vi "final_control_mk6_022725.vi"() -> ()   [LabVIEW 2023]
doc: "Simplified example program for initializing the COM port, determining the data frame of up to 26 Alicats, acquiring the data of the same number of Alicats, displaying the data of the one with the selected unit ID, and writing a setpoint to the same selected unit ID.\n\nThis is a slightly more feature rich version of the Alicat Simplified Driver Example, and contains an example of a method for interfacing with up to 26 Alicats on a single COM port by means of for loops with shift registers to handle sequential commands to each included Alicat. This also contains a method to write a setpoint to the same selected unit.\n\nIf coding for multiple Alicats on a single COM port without the use of for loops with shift registers, ensure that each Alicat command is executed sequentially. Alicat's RS-232/485 does not work if multiple devices are responding simultaneously."
uses:
  <vilib>/Platform/TimedLoop/XDataNode/timing_clust.ctl
  <vilib>/Platform/TimedLoop/XDataNode/nitl_modes.ctl
  <vilib>/Platform/TimedLoop/XDataNode/wakeup.ctl
  <vilib>/DAQmx/write.llb/DAQmx Write (Analog 1D DBL NChan 1Samp).vi
  <extravilib>/ChannelInstances/Tag-bool/Read With Abort.vi
  <extravilib>/ChannelInstances/Tag-bool/Write With Abort.vi
  <vilib>/Utility/file.llb/Write Delimited Spreadsheet (string).vi
  <extravilib>/ChannelInstances/Tag-bool/Instantiate.vi
  <vilib>/Utility/file.llb/Read Delimited Spreadsheet (DBL).vi
  <extravilib>/ChannelInstances/Tag-bool/EndpointRead.vi
  <vilib>/DAQmx/miscellaneous.llb/DAQmx Fill In Error Info.vi
  <extravilib>/ChannelInstances/Tag-bool/Endpoint.vi
  <vilib>/platform/TimedLoop/XDataNode/XDataNode.xnode
  <vilib>/DAQmx/read.llb/DAQmx Read (Analog 1D DBL 1Chan NSamp).vi
  <vilib>/Platform/TimedLoop/XDataNode/XDNodeRunTimeDep.lvlib
  <extravilib>/ChannelInstances/Tag-bool.lvlib
panel:
  in  "Tab Control":enum32{"Page 1", "Page 2"}(tab)
  in  "COM Port Settings":T1={"Baud Rate"=enum."19200", "VISA Sesssion In"="MassFlowControllers"}
  out "Range Exceeded":bool
  out "Error Present":bool
  out "Error Text":string
  out "Elapsed Time [ms]\n(all units)":dbl caption="Elapsed Time (s)"
  in  "Minimum time between \nreadings [ms] (all units)":u32
  in  "Device ID's \nto Include:":T2={"A"=TRUE, "B"=TRUE, "C"=TRUE, "D"=TRUE, "E"=TRUE, "F"=TRUE, "G"=FALSE, "H"=FALSE, "I"=FALSE, "J"=FALSE, "K"=FALSE, "L"=FALSE, "M"=FALSE, "N"=FALSE, "O"=FALSE, "P"=FALSE, "Q"=FALSE, "R"=FALSE, "S"=FALSE, "T"=FALSE, "U"=FALSE, "V"=FALSE, "W"=FALSE, "X"=FALSE, "Y"=FALSE, "Z"=FALSE}
  out "Active Device":u16(ring) items=["A", "B", "C", "D", "E", "F"]
  out "Meas. Data (for active device)":T3
  in  "Write File":path
  in  "Hold Time [min]":dbl=17.0 min=17.0
  out "Global Start Time":i64
  out "N":i32
  out "Iteration Duration":i64
  in  "Read File":path
  in  "End Program":bool
  in  "Start From:":i32
  out "len_SP":i32
  out "Setpoints":dbl[][](array[numeric])=[[4.2, 3.3], [69.0, 4.2]]
  out "Z":dbl[](array[numeric])
  out "ASP":dbl
  out "BSP":dbl
  out "CSP":dbl
  out "DSP":dbl
  out "ESP":dbl
  out "FSP":dbl
  out "N_i_read":dbl
  out "N_read":i32
  out "read count":dbl=2.0
  out "T_SCh":string[](array[string])
  out "Iter_#":string
  out "V_D":string
  out "V_H":string
  out "Iter_Duration":string
  out "all rows":dbl[][](array[numeric])
  # "Totalizer Timer"
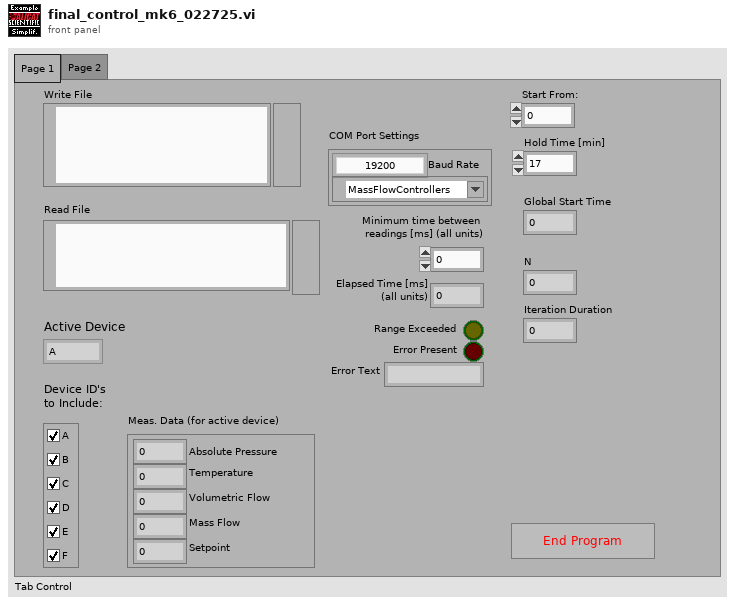
[diagram p1: front panel]
types:
  T1 = cluster{"Baud Rate":enum8{"2400", "9600", "19200", "38400", "57600", "115200", "Unknown"}, "VISA Sesssion In":refnum<visa-resource-name>}
  T2 = cluster{"A":bool, "B":bool, "C":bool, "D":bool, "E":bool, "F":bool, "G":bool, "H":bool, "I":bool, "J":bool, "K":bool, "L":bool, "M":bool, "N":bool, "O":bool, "P":bool, "Q":bool, "R":bool, "S":bool, "T":bool, "U":bool, "V":bool, "W":bool, "X":bool, "Y":bool, "Z":bool}
  T3 = cluster{"Absolute Pressure":dbl, "Gauge/Diff. Pressure":dbl, "Barometric Pressure":dbl, "Temperature":dbl, "Volumetric Flow":dbl, "Mass Flow":dbl, "Setpoint":dbl, "Valve Drive":dbl, "Totalizer":dbl, "[hr]":dbl, "[min]":dbl, "[sec]":dbl, "Totalizer Average Flow":dbl, "Totalizer Peak Flow":dbl, "Gas selected":string}
  T4 = cluster{"Unit ID":string, "Baud Rate":enum8{"2400", "9600", "19200", "38400", "57600", "115200", "Unknown"}, "VISA Sesssion In":refnum<visa-resource-name>}
  T5 = typedef "XDNodeRunTimeDep.lvlib/timing_clust.ctl" = cluster{"Expected End [f-1]":u64, "Actual End [f-1]":u64, "Finished Late? [f-1]":bool, "Expected End [i-1]":u64, "Actual End [i-1]":u64, "Finished Late? [i-1]":bool, "Expected Start [i]":u64, "Actual Start [i]":u64, "Expected Start [f]":u64, "Actual Start [f]":u64, "Source Name":string, "Structure Name":string, "Period":i64, "Deadline":i64, "Offset":i64, "Start":i64, "Priority":i32, "Timeout":i32, "Mode":T6, "Wakeup Reason":T7, "Error":errorcluster, "Source Type":string, "Secondary Source Type":string, "Global End Time":u64, "Global Start Time":u64, "Frame Duration":u64, "Iteration Duration":u64, "Assigned CPU":i32, "I/O Scan Engine Mode":u32}
  T6 = typedef "XDNodeRunTimeDep.lvlib/nitl_modes.ctl" = enum32{"No Change", "Process missed periods, maintain original phase", "Discard missed periods, maintain original phase", "Process missed periods, ignore original phase", "Discard missed periods, ignore original phase"}
  T7 = typedef "XDNodeRunTimeDep.lvlib/wakeup.ctl" = enum32{"Normal", "Aborted", "Asynchronous wakeup", "Timing source error", "Timed loop error", "Timeout"}
  T8 = typedef "Tag-bool.lvlib/))Channel.ctl" = refnum<queue>
  T9 = enum8{"2400", "9600", "19200", "38400", "57600", "115200", "Unknown"}
  T10 = cluster{"Absolute Pressure":bool, "Gauge/Diff. Pressure":bool, "Barometric Pressure":bool, "Temperature":bool, "Volumetric":bool, "Mass":bool, "Setpoint":bool, "Valve Drive":bool, "Totalizer":bool, "Totalizer Timer":bool, "Totalizer Average Flow":bool, "Totalizer Peak Flow":bool, "Gas Selected":bool, "Tot. Timer Format":u16}
  T11 = cluster{"Controller Full Scale":dbl, "Controller Select":u16, "Control Range":enum16{"Normal", "Inverted", "Bidirectional", "Unknown"}}
  T12 = cluster{"Controller Full Scale":dbl, "Controller Select":u16, "Control Range":enum16{"Normal", "Inverted", "Bidirectional", "Unknown"}}[]
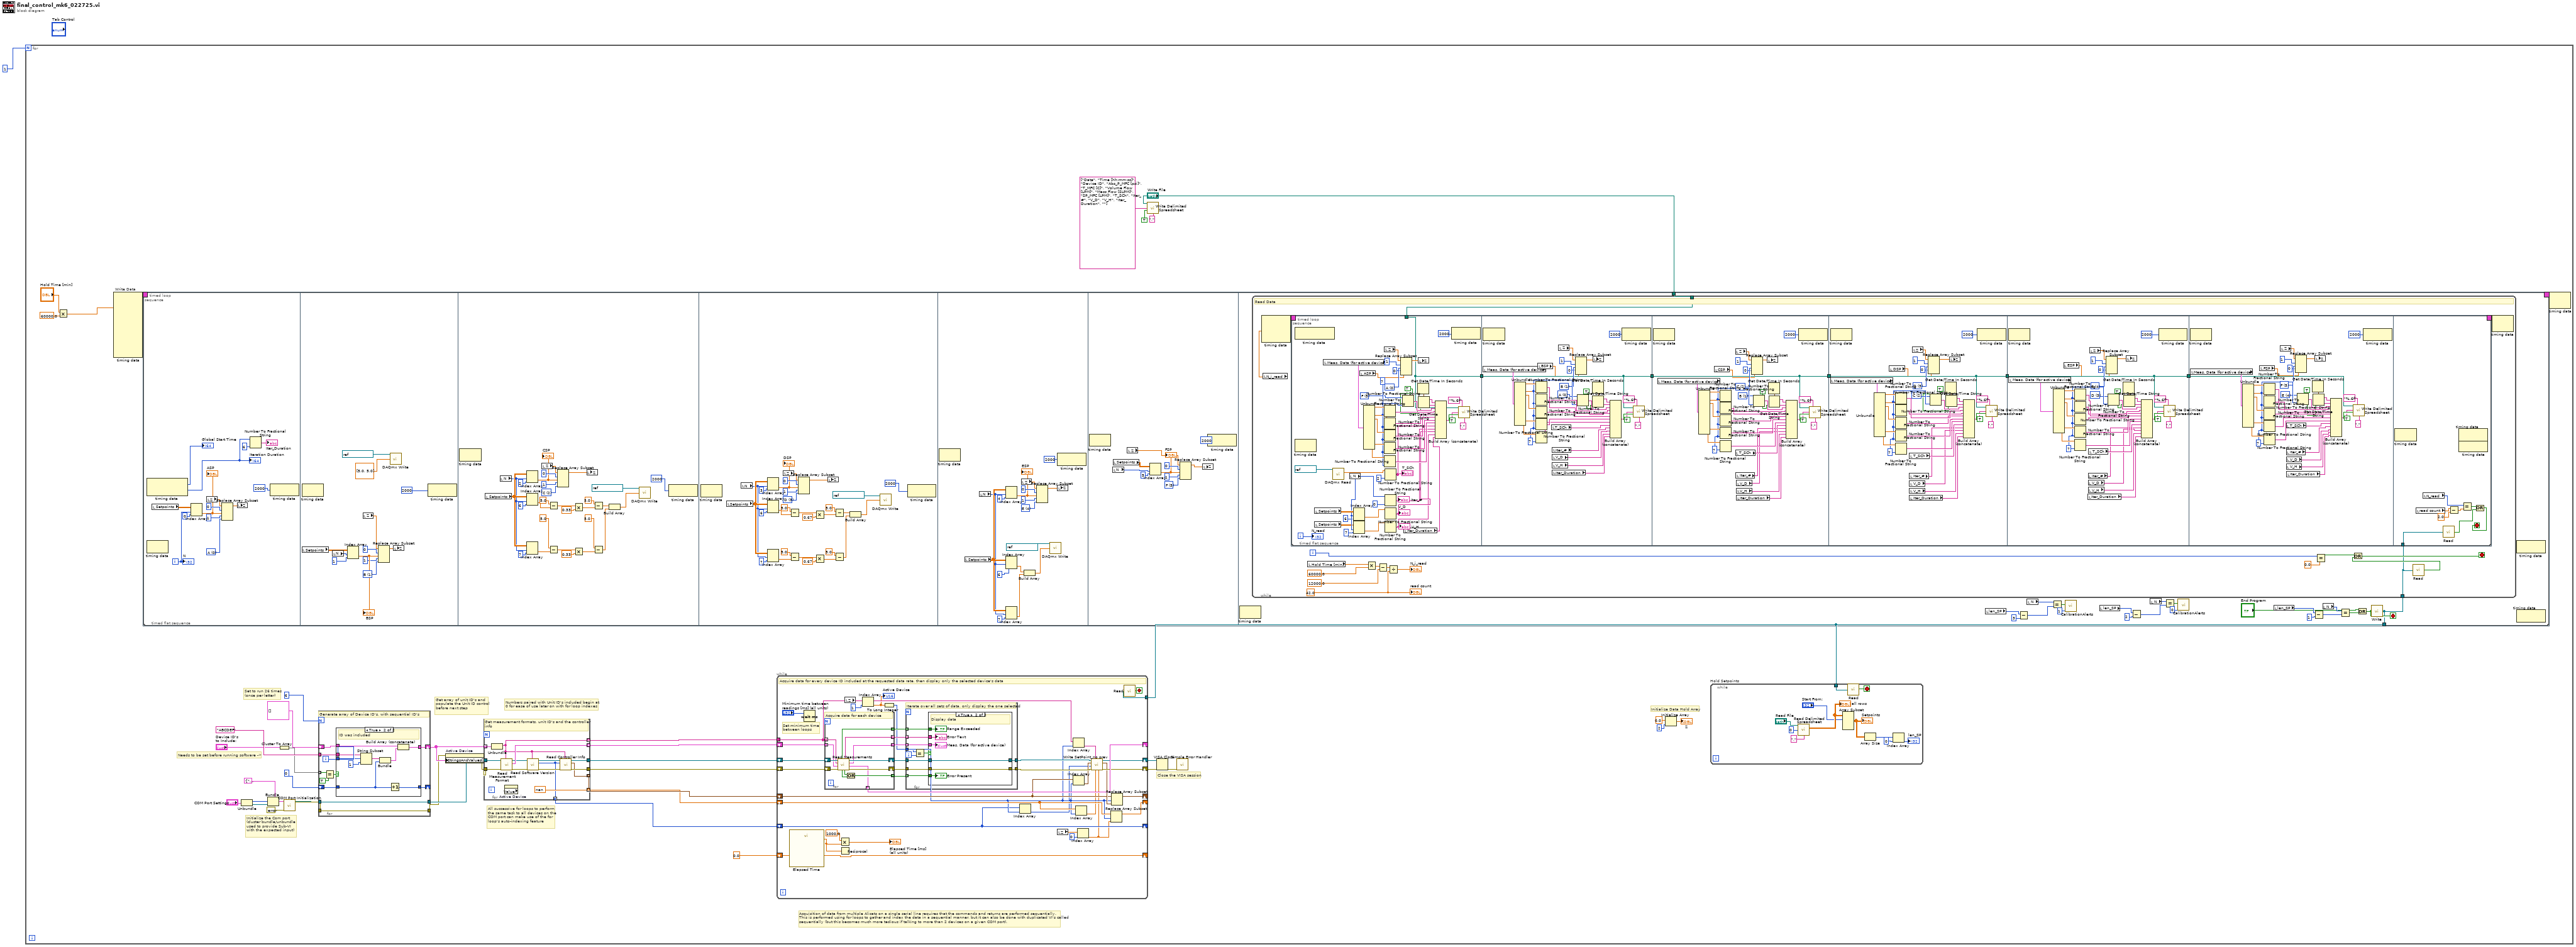
[diagram p0: block diagram]
diagram:
  n1 = for {
    N: 1 -> [_]
    # "Initialize Data Hold Array"
    # "All successive for loops to perform\nthe same task to all devices on the\nCOM port can make use of the for\nloop's auto-indexing feature"
    # "Set to run 26 times\n(once per letter)"
    # "Acquisition of data from multiple Alicats on a single serial line requires that the commands and returns are performed sequentially.\nThis is performed using for loops to gather and index the data in a sequential manner, but it can also be done with duplicated VI's called\nsequentially (but this becomes much more tedious if talking to more than 2 devices on a given COM port)."
    # "Numbers paired with Unit ID's included begin at\n0 for ease of use later on with for loop indexes"
    # "Get array of unit ID's and populate the Unit ID control before next step"
    # "Needs to be set before running software ->"
    # "Close the VISA session"
    # "Initialize the Com port\n(cluster bundle/unbundle\nused to provide Sub-VI \nwith the expected input)"
    n2 = Multiply(x="Hold Time [min]", y=60000.0) -> (x*y=w2:dbl)
    n3 = node-c288(w2) -> (w43:T5)  [unwired: 9 in]
    n4 = timed-loop "Write Data" {
      timing: w43 -> [_]
      timing-out: [_] -> w42
      tunnel: [w56] -> w9
      tunnel: "Write File" -> [w55]
      i -> [w70]
      stop <- w210 stop-if-true
      n5 = timed-sequence {
        timing: _ -> [_]
        timing-out: _ -> [_]
        tunnel: [w58] -> w56
        tunnel: w55 -> [w57]
        n6 = timed-flat-sequence {
          tunnel: [w205] -> w58
          tunnel: w57 -> [w206]
          frame #0 {
            w63 = u16 0 items=["A", "B", "C", "D", "E", "F"]
            n7 = node-c288() -> (→"Global Start Time":i64, w62:i64)  [unwired: 1 in]
            "Iteration Duration" <- w62
            n8 = local read "Setpoints"() -> (w72:dbl[][])
            n9 = Index Array(array=w72, index (row)=w70, index (col)=0 ("index (row)")) -> (element=w68:dbl)
            "ASP" <- w68
            n10 = local read "Z"() -> (w66:dbl[])
            n11 = Replace Array Subset(array=w66, new element #1=w68, index #1=0 ("index"), new element #2=w63, index #2=1 ("index")) -> (w67:dbl[])
            n12 = local write "Z"(w67) -> ()
            n13 = Number To Fractional String(number=w62, precision (6)=i16 6) -> (F-format string=→"Iter_Duration":string)  [unwired: 2 in]
            n14 = node-c288(i64 2000 ("Start")) -> ()  [unwired: 1 out]
            "N" <- w70
          }
          frame #1 {
            w81 = u16 1 items=["A", "B", "C", "D", "E", "F"]
            n15 = node-c288() -> ()  [unwired: 1 in, 1 out]
            n16 = local read "Setpoints"() -> (w89:dbl[][])
            n17 = local read "N"() -> (w82:i32)
            n18 = Index Array(array=w89, index (row)=w82, index (col)=1 ("index (row)")) -> (element=w86:dbl)
            "BSP" <- w86
            n19 = local read "Z"() -> (w84:dbl[])
            n20 = Replace Array Subset(array=w84, new element #1=w86, index #1=0 ("index"), new element #2=w81, index #2=1 ("index")) -> (w85:dbl[])
            n21 = call-poly <vilib>:"DAQmx Write.vi"("task/channels in"=refnum<k21> "Valve_cont", "data"=dbl[] [5.0, 5.0]) -> ()  [unwired: 11 in, 3 out]
            n22 = local write "Z"(w85) -> ()
            n23 = node-c288(i64 2000 ("Start")) -> ()  [unwired: 1 out]
          }
          frame #2 {
            w115 = u16 2 items=["A", "B", "C", "D", "E", "F"]
            n24 = node-c288() -> ()  [unwired: 1 in, 1 out]
            n25 = local read "Setpoints"() -> (w98:dbl[][])
            n26 = local read "N"() -> (w97:i32)
            n27 = Index Array(array=w98, index (row)=w97, index (col)=2 ("index (row)")) -> (element=w119:dbl)
            "CSP" <- w119
            n28 = Index Array(array=w98, index (row)=w97, index (col)=6 ("disabled index (col)")) -> (element=w96:dbl)
            n29 = Index Array(array=w98, index (row)=w97, index (col)=7 ("disabled index (col)")) -> (element=w95:dbl)
            n30 = local read "Z"() -> (w117:dbl[])
            n31 = Subtract(x=5.0, y=w96) -> (x-y=w112:dbl)
            n32 = Subtract(x=5.0, y=w95) -> (x-y=w107:dbl)
            n33 = Replace Array Subset(array=w117, new element #1=w119, index #1=0 ("index"), new element #2=w115, index #2=1 ("index")) -> (w118:dbl[])
            n34 = Multiply(x=w112, y=0.33) -> (x*y=w110:dbl)
            n35 = Multiply(x=w107, y=0.33) -> (x*y=w105:dbl)
            n36 = local write "Z"(w118) -> ()
            n37 = Subtract(x=5.0, y=w110) -> (x-y=w100:dbl)
            n38 = Subtract(x=5.0, y=w105) -> (x-y=w101:dbl)
            n39 = Build Array(w100, w101) -> (w99:dbl[])
            n40 = call-poly <vilib>:"DAQmx Write.vi"("task/channels in"=refnum<k21> "Valve_cont", "data"=w99) -> ()  [unwired: 11 in, 3 out]
            n41 = node-c288(i64 2000 ("Start")) -> ()  [unwired: 1 out]
          }
          frame #3 {
            w147 = u16 3 items=["A", "B", "C", "D", "E", "F"]
            n42 = node-c288() -> ()  [unwired: 1 in, 1 out]
            n43 = local read "Setpoints"() -> (w130:dbl[][])
            n44 = local read "N"() -> (w129:i32)
            n45 = Index Array(array=w130, index (row)=w129, index (col)=3 ("index (row)")) -> (element=w151:dbl)
            "DSP" <- w151
            n46 = Index Array(array=w130, index (row)=w129, index (col)=6 ("disabled index (col)")) -> (element=w128:dbl)
            n47 = Index Array(array=w130, index (row)=w129, index (col)=7 ("disabled index (col)")) -> (element=w127:dbl)
            n48 = local read "Z"() -> (w149:dbl[])
            n49 = Subtract(x=5.0, y=w128) -> (x-y=w144:dbl)
            n50 = Subtract(x=5.0, y=w127) -> (x-y=w139:dbl)
            n51 = Replace Array Subset(array=w149, new element #1=w151, index #1=0 ("index"), new element #2=w147, index #2=1 ("index")) -> (w150:dbl[])
            n52 = Multiply(x=w144, y=0.67) -> (x*y=w142:dbl)
            n53 = Multiply(x=w139, y=0.67) -> (x*y=w137:dbl)
            n54 = local write "Z"(w150) -> ()
            n55 = Subtract(x=5.0, y=w142) -> (x-y=w132:dbl)
            n56 = Subtract(x=5.0, y=w137) -> (x-y=w133:dbl)
            n57 = Build Array(w132, w133) -> (w131:dbl[])
            n58 = call-poly <vilib>:"DAQmx Write.vi"("task/channels in"=refnum<k21> "Valve_cont", "data"=w131) -> ()  [unwired: 11 in, 3 out]
            n59 = node-c288(i64 2000 ("Start")) -> ()  [unwired: 1 out]
          }
          frame #4 {
            w168 = u16 4 items=["A", "B", "C", "D", "E", "F"]
            n60 = node-c288() -> ()  [unwired: 1 in, 1 out]
            n61 = local read "Setpoints"() -> (w162:dbl[][])
            n62 = local read "N"() -> (w161:i32)
            n63 = Index Array(array=w162, index (row)=w161, index (col)=4 ("index (row)")) -> (element=w172:dbl)
            "ESP" <- w172
            n64 = Index Array(array=w162, index (row)=w161, index (col)=6 ("disabled index (col)")) -> (element=w164:dbl)
            n65 = Index Array(array=w162, index (row)=w161, index (col)=7 ("disabled index (col)")) -> (element=w163:dbl)
            n66 = local read "Z"() -> (w170:dbl[])
            n67 = Build Array(w164, w163) -> (w160:dbl[])
            n68 = Replace Array Subset(array=w170, new element #1=w172, index #1=0 ("index"), new element #2=w168, index #2=1 ("index")) -> (w171:dbl[])
            n69 = call-poly <vilib>:"DAQmx Write.vi"("task/channels in"=refnum<k21> "Valve_cont", "data"=w160) -> ()  [unwired: 11 in, 3 out]
            n70 = local write "Z"(w171) -> ()
            n71 = node-c288(i64 2000 ("Start")) -> ()  [unwired: 1 out]
          }
          frame #5 {
            w182 = u16 5 items=["A", "B", "C", "D", "E", "F"]
            n72 = node-c288() -> ()  [unwired: 1 in, 1 out]
            n73 = local read "N"() -> (w180:i32)
            n74 = local read "Setpoints"() -> (w185:dbl[][])
            n75 = local read "Z"() -> (w184:dbl[])
            n76 = Index Array(array=w185, index (row)=w180, index (col)=5 ("index (row)")) -> (element=w181:dbl)
            "FSP" <- w181
            n77 = Replace Array Subset(array=w184, new element #1=w181, index #1=0 ("index"), new element #2=w182, index #2=1 ("index")) -> (w183:dbl[])
            n78 = local write "Z"(w183) -> ()
            n79 = node-c288(i64 2000 ("Start")) -> ()  [unwired: 1 out]
          }
          frame #6 {
            n80 = node-c288() -> ()  [unwired: 1 in, 1 out]
            n81 = local read "len_SP"() -> (w194:i32)
            n82 = Subtract(x=w194, y=3) -> (x-y=w196:i32)
            n83 = local read "N"() -> (w195:i32)
            n84 = Equal?(x=w195, y=w196) -> (x = y?=w197:bool)
            n85 = call "CalibrationAlerts.vi"("Alert Type (0)"=1, "Trigger"=w197) -> ()  [unwired: 10 in]
            n86 = local read "len_SP"() -> (w200:i32)
            n87 = Subtract(x=w200, y=2) -> (x-y=w199:i32)
            n88 = local read "N"() -> (w204:i32)
            n89 = Equal?(x=w204, y=w199) -> (x = y?=w202:bool)
            n90 = call "CalibrationAlerts.vi"("Alert Type (0)"=0, "Trigger"=w202) -> ()  [unwired: 10 in]
            n91 = local read "len_SP"() -> (w209:i32)
            n92 = Subtract(x=w209, y=1) -> (x-y=w212:i32)
            n93 = local read "N"() -> (w208:i32)
            n94 = Equal?(x=w208, y=w212) -> (x = y?=w211:bool)
            n95 = Or(x="End Program", y=w211) -> (x .or. y?=w210:bool)
            n96 = call <extravilib>:"Write.vi"("element"=w210) -> ("channel"=w205:T8)  [unwired: 1 out]
            n97 = while {
              tunnel: w206 -> [w228]
              tunnel: w205 -> [w214]
              i -> [w224]
              stop <- w223 stop-if-true
              w217 = 42.0 ("y")
              # "Read Data"
              n98 = local read "N_i_read"() -> (w222:dbl)
              n99 = node-c288(w222) -> (w230:T5)  [unwired: 2 in]
              n100 = timed-loop {
                timing: w230 -> [_]
                timing-out: [_] -> w229
                tunnel: w228 -> [w232]
                tunnel: w214 -> [w231]
                i -> [w258]
                stop <- w487 stop-if-true
                n101 = timed-sequence {
                  timing: _ -> [_]
                  timing-out: _ -> [_]
                  tunnel: w232 -> [w239]
                  tunnel: w231 -> [w233]
                  n102 = timed-flat-sequence {
                    tunnel: w239 -> [w261]
                    tunnel: [w261] -> w238
                    tunnel: w238 -> [w300]
                    tunnel: [w300] -> w237
                    tunnel: w237 -> [w339]
                    tunnel: [w339] -> w236
                    tunnel: w236 -> [w378]
                    tunnel: [w378] -> w235
                    tunnel: w235 -> [w417]
                    tunnel: [w417] -> w234
                    tunnel: w234 -> [w457]
                    tunnel: w233 -> [w489]
                    frame #0 {
                      w257 = u16 5 items=["A", "B", "C", "D", "E", "F"]
                      w264 = u16 0 items=["A", "B", "C", "D", "E", "F"]
                      w265 = i16 7 ("precision (6)")
                      n103 = node-c288() -> ()  [unwired: 1 in, 1 out]
                      n104 = local read "Setpoints"() -> (w251:dbl[][])
                      n105 = local read "Setpoints"() -> (w247:dbl[][])
                      n106 = local read "Meas. Data (for active device)"() -> (w272:T3)
                      n107 = call-poly <vilib>:"DAQmx Read.vi"("task/channels in"=refnum<k21> "T_SCh") -> ("data"=w255:dbl[])  [unwired: 12 in, 2 out]
                      n108 = local read "N"() -> (w248:i32)
                      n109 = Index Array(array=w251, index (row)=w248, index (col)=6 ("disabled index (col)")) -> (element=w250:dbl)
                      n110 = Index Array(array=w247, index (row)=w248, index (col)=7 ("disabled index (col)")) -> (element=w249:dbl)
                      n111 = local read "ASP"() -> (w259:dbl)
                      n112 = Unbundle(w272) -> ("Absolute Pressure"=w285:dbl, "Temperature"=w281:dbl, "Volumetric Flow"=w271:dbl, "Mass Flow"=w282:dbl, "Setpoint"=w283:dbl)  [unwired: 10 out]
                      n113 = local read "Z"() -> (w268:dbl[])
                      n114 = Number To Fractional String(number=w285, precision (6)=w265) -> (F-format string=w280:string)  [unwired: 2 in]
                      n115 = Number To Fractional String(number=w281, precision (6)=w265) -> (F-format string=w279:string)  [unwired: 2 in]
                      n116 = Number To Fractional String(number=w271, precision (6)=w265) -> (F-format string=w278:string)  [unwired: 2 in]
                      n117 = Number To Fractional String(number=w282, precision (6)=w265) -> (F-format string=w277:string)  [unwired: 2 in]
                      n118 = Number To Fractional String(number=w283, precision (6)=w265) -> (F-format string=w276:string)  [unwired: 2 in]
                      n119 = Number To Fractional String(number=w255, precision (6)=i16 2) -> (F-format string=w254:string[])  [unwired: 2 in]
                      "T_SCh" <- w254
                      n120 = Number To Fractional String(number=w248, precision (6)=i16 0) -> (F-format string=w243:string)  [unwired: 2 in]
                      "Iter_#" <- w243
                      n121 = Number To Fractional String(number=w250) -> (F-format string=w242:string)  [unwired: 3 in]
                      "V_D" <- w242
                      n122 = Number To Fractional String(number=w249) -> (F-format string=w241:string)  [unwired: 3 in]
                      "V_H" <- w241
                      n123 = Replace Array Subset(array=w268, new element #1=w264, index #1=1 ("index"), new element #2=w259, index #2=0 ("index")) -> (w266:dbl[])
                      n124 = Number To Fractional String(number=w257, precision (6)=w265) -> (F-format string=w284:string)  [unwired: 2 in]
                      n125 = local read "Iter_Duration"() -> (w240:string)
                      n126 = Get Date/Time In Seconds() -> (seconds since 1Jan1904=w270:timestamp)
                      n127 = Get Date/Time String(seconds (now)=w270, want seconds? (F)=TRUE) -> (date string=w269:string, time string=w286:string)  [unwired: 1 in]
                      n128 = local write "Z"(w266) -> ()
                      n129 = Build Array (concatenate)(w269, w286, w284, w280, w279, w278, w277, w276, w254, w243, w242, w241, w240) -> (w273:string[])
                      n130 = node-c288(i64 2000 ("Start")) -> ()  [unwired: 1 out]
                      n131 = call-poly <vilib>:"Write Delimited Spreadsheet.vi"("file path (dialog if empty)"=w261, "format (%s)"="%.6f" ("format (%.3f)"), "1D data"=w273, "append to file? (new file:F)"=TRUE, "delimiter (\\t)"="," ("delimiter (\\t)")) -> ()  [unwired: 9 in, 2 out]
                      "N_read" <- w258
                    }
                    frame #1 {
                      w297 = u16 0 items=["A", "B", "C", "D", "E", "F"]
                      w306 = u16 1 items=["A", "B", "C", "D", "E", "F"]
                      w307 = i16 7 ("precision (6)")
                      n132 = node-c288() -> ()  [unwired: 1 in, 1 out]
                      n133 = local read "Meas. Data (for active device)"() -> (w304:T3)
                      n134 = Unbundle(w304) -> ("Absolute Pressure"=w324:dbl, "Temperature"=w320:dbl, "Volumetric Flow"=w311:dbl, "Mass Flow"=w321:dbl, "Setpoint"=w322:dbl)  [unwired: 10 out]
                      n135 = Number To Fractional String(number=w324, precision (6)=w307) -> (F-format string=w319:string)  [unwired: 2 in]
                      n136 = Number To Fractional String(number=w320, precision (6)=w307) -> (F-format string=w318:string)  [unwired: 2 in]
                      n137 = Number To Fractional String(number=w311, precision (6)=w307) -> (F-format string=w317:string)  [unwired: 2 in]
                      n138 = Number To Fractional String(number=w321, precision (6)=w307) -> (F-format string=w316:string)  [unwired: 2 in]
                      n139 = Number To Fractional String(number=w322, precision (6)=w307) -> (F-format string=w315:string)  [unwired: 2 in]
                      n140 = local read "BSP"() -> (w298:dbl)
                      n141 = local read "T_SCh"() -> (w296:string[])
                      n142 = local read "Iter_#"() -> (w294:string)
                      n143 = local read "V_D"() -> (w293:string)
                      n144 = local read "V_H"() -> (w292:string)
                      n145 = local read "Iter_Duration"() -> (w291:string)
                      n146 = local read "Z"() -> (w303:dbl[])
                      n147 = Replace Array Subset(array=w303, new element #1=w306, index #1=1 ("index"), new element #2=w298, index #2=0 ("index")) -> (w302:dbl[])
                      n148 = Number To Fractional String(number=w297, precision (6)=w307) -> (F-format string=w323:string)  [unwired: 2 in]
                      n149 = Get Date/Time In Seconds() -> (seconds since 1Jan1904=w310:timestamp)
                      n150 = Get Date/Time String(seconds (now)=w310, want seconds? (F)=TRUE) -> (date string=w309:string, time string=w325:string)  [unwired: 1 in]
                      n151 = local write "Z"(w302) -> ()
                      n152 = Build Array (concatenate)(w309, w325, w323, w319, w318, w317, w316, w315, w296, w294, w293, w292, w291) -> (w312:string[])
                      n153 = node-c288(i64 2000 ("Start")) -> ()  [unwired: 1 out]
                      n154 = call-poly <vilib>:"Write Delimited Spreadsheet.vi"("file path (dialog if empty)"=w300, "format (%s)"="%.6f" ("format (%.3f)"), "1D data"=w312, "append to file? (new file:F)"=TRUE, "delimiter (\\t)"="," ("delimiter (\\t)")) -> ()  [unwired: 9 in, 2 out]
                    }
                    frame #2 {
                      w336 = u16 1 items=["A", "B", "C", "D", "E", "F"]
                      w345 = u16 2 items=["A", "B", "C", "D", "E", "F"]
                      w346 = i16 7 ("precision (6)")
                      n155 = node-c288() -> ()  [unwired: 1 in, 1 out]
                      n156 = local read "Meas. Data (for active device)"() -> (w341:T3)
                      n157 = Unbundle(w341) -> ("Absolute Pressure"=w363:dbl, "Temperature"=w359:dbl, "Volumetric Flow"=w350:dbl, "Mass Flow"=w360:dbl, "Setpoint"=w361:dbl)  [unwired: 10 out]
                      n158 = local read "CSP"() -> (w337:dbl)
                      n159 = Number To Fractional String(number=w363, precision (6)=w346) -> (F-format string=w358:string)  [unwired: 2 in]
                      n160 = Number To Fractional String(number=w359, precision (6)=w346) -> (F-format string=w357:string)  [unwired: 2 in]
                      n161 = Number To Fractional String(number=w350, precision (6)=w346) -> (F-format string=w356:string)  [unwired: 2 in]
                      n162 = Number To Fractional String(number=w360, precision (6)=w346) -> (F-format string=w355:string)  [unwired: 2 in]
                      n163 = Number To Fractional String(number=w361, precision (6)=w346) -> (F-format string=w354:string)  [unwired: 2 in]
                      n164 = local read "Z"() -> (w343:dbl[])
                      n165 = local read "T_SCh"() -> (w335:string[])
                      n166 = local read "Iter_#"() -> (w333:string)
                      n167 = local read "V_D"() -> (w332:string)
                      n168 = local read "V_H"() -> (w331:string)
                      n169 = local read "Iter_Duration"() -> (w330:string)
                      n170 = Replace Array Subset(array=w343, new element #1=w345, index #1=1 ("index"), new element #2=w337, index #2=0 ("index")) -> (w342:dbl[])
                      n171 = Number To Fractional String(number=w336, precision (6)=w346) -> (F-format string=w362:string)  [unwired: 2 in]
                      n172 = local write "Z"(w342) -> ()
                      n173 = Get Date/Time In Seconds() -> (seconds since 1Jan1904=w349:timestamp)
                      n174 = Get Date/Time String(seconds (now)=w349, want seconds? (F)=TRUE) -> (date string=w348:string, time string=w364:string)  [unwired: 1 in]
                      n175 = Build Array (concatenate)(w348, w364, w362, w358, w357, w356, w355, w354, w335, w333, w332, w331, w330) -> (w351:string[])
                      n176 = node-c288(i64 2000 ("Start")) -> ()  [unwired: 1 out]
                      n177 = call-poly <vilib>:"Write Delimited Spreadsheet.vi"("file path (dialog if empty)"=w339, "format (%s)"="%.6f" ("format (%.3f)"), "1D data"=w351, "append to file? (new file:F)"=TRUE, "delimiter (\\t)"="," ("delimiter (\\t)")) -> ()  [unwired: 9 in, 2 out]
                    }
                    frame #3 {
                      w375 = u16 2 items=["A", "B", "C", "D", "E", "F"]
                      w384 = u16 3 items=["A", "B", "C", "D", "E", "F"]
                      w385 = i16 7 ("precision (6)")
                      n178 = node-c288() -> ()  [unwired: 1 in, 1 out]
                      n179 = local read "Meas. Data (for active device)"() -> (w382:T3)
                      n180 = Unbundle(w382) -> ("Absolute Pressure"=w402:dbl, "Temperature"=w398:dbl, "Volumetric Flow"=w389:dbl, "Mass Flow"=w399:dbl, "Setpoint"=w400:dbl)  [unwired: 10 out]
                      n181 = local read "DSP"() -> (w376:dbl)
                      n182 = Number To Fractional String(number=w402, precision (6)=w385) -> (F-format string=w397:string)  [unwired: 2 in]
                      n183 = Number To Fractional String(number=w398, precision (6)=w385) -> (F-format string=w396:string)  [unwired: 2 in]
                      n184 = Number To Fractional String(number=w389, precision (6)=w385) -> (F-format string=w395:string)  [unwired: 2 in]
                      n185 = Number To Fractional String(number=w399, precision (6)=w385) -> (F-format string=w394:string)  [unwired: 2 in]
                      n186 = Number To Fractional String(number=w400, precision (6)=w385) -> (F-format string=w393:string)  [unwired: 2 in]
                      n187 = local read "T_SCh"() -> (w374:string[])
                      n188 = local read "Iter_#"() -> (w372:string)
                      n189 = local read "V_D"() -> (w371:string)
                      n190 = local read "V_H"() -> (w370:string)
                      n191 = local read "Iter_Duration"() -> (w369:string)
                      n192 = local read "Z"() -> (w381:dbl[])
                      n193 = Replace Array Subset(array=w381, new element #1=w384, index #1=1 ("index"), new element #2=w376, index #2=0 ("index")) -> (w380:dbl[])
                      n194 = Number To Fractional String(number=w375, precision (6)=w385) -> (F-format string=w401:string)  [unwired: 2 in]
                      n195 = Get Date/Time In Seconds() -> (seconds since 1Jan1904=w388:timestamp)
                      n196 = Get Date/Time String(seconds (now)=w388, want seconds? (F)=TRUE) -> (date string=w387:string, time string=w403:string)  [unwired: 1 in]
                      n197 = local write "Z"(w380) -> ()
                      n198 = Build Array (concatenate)(w387, w403, w401, w397, w396, w395, w394, w393, w374, w372, w371, w370, w369) -> (w390:string[])
                      n199 = node-c288(i64 2000 ("Start")) -> ()  [unwired: 1 out]
                      n200 = call-poly <vilib>:"Write Delimited Spreadsheet.vi"("file path (dialog if empty)"=w378, "format (%s)"="%.6f" ("format (%.3f)"), "1D data"=w390, "append to file? (new file:F)"=TRUE, "delimiter (\\t)"="," ("delimiter (\\t)")) -> ()  [unwired: 9 in, 2 out]
                    }
                    frame #4 {
                      w414 = u16 3 items=["A", "B", "C", "D", "E", "F"]
                      w423 = u16 4 items=["A", "B", "C", "D", "E", "F"]
                      w424 = i16 7 ("precision (6)")
                      n201 = node-c288() -> ()  [unwired: 1 in, 1 out]
                      n202 = local read "Meas. Data (for active device)"() -> (w421:T3)
                      n203 = Unbundle(w421) -> ("Absolute Pressure"=w441:dbl, "Temperature"=w437:dbl, "Volumetric Flow"=w428:dbl, "Mass Flow"=w438:dbl, "Setpoint"=w439:dbl)  [unwired: 10 out]
                      n204 = local read "ESP"() -> (w415:dbl)
                      n205 = Number To Fractional String(number=w441, precision (6)=w424) -> (F-format string=w436:string)  [unwired: 2 in]
                      n206 = Number To Fractional String(number=w437, precision (6)=w424) -> (F-format string=w435:string)  [unwired: 2 in]
                      n207 = Number To Fractional String(number=w428, precision (6)=w424) -> (F-format string=w434:string)  [unwired: 2 in]
                      n208 = Number To Fractional String(number=w438, precision (6)=w424) -> (F-format string=w433:string)  [unwired: 2 in]
                      n209 = Number To Fractional String(number=w439, precision (6)=w424) -> (F-format string=w432:string)  [unwired: 2 in]
                      n210 = local read "Iter_Duration"() -> (w408:string)
                      n211 = local read "Iter_#"() -> (w411:string)
                      n212 = local read "V_D"() -> (w410:string)
                      n213 = local read "V_H"() -> (w409:string)
                      n214 = local read "T_SCh"() -> (w413:string[])
                      n215 = local read "Z"() -> (w420:dbl[])
                      n216 = Replace Array Subset(array=w420, new element #1=w423, index #1=1 ("index"), new element #2=w415, index #2=0 ("index")) -> (w419:dbl[])
                      n217 = Number To Fractional String(number=w414, precision (6)=w424) -> (F-format string=w440:string)  [unwired: 2 in]
                      n218 = Get Date/Time In Seconds() -> (seconds since 1Jan1904=w427:timestamp)
                      n219 = Get Date/Time String(seconds (now)=w427, want seconds? (F)=TRUE) -> (date string=w426:string, time string=w442:string)  [unwired: 1 in]
                      n220 = local write "Z"(w419) -> ()
                      n221 = Build Array (concatenate)(w426, w442, w440, w436, w435, w434, w433, w432, w413, w411, w410, w409, w408) -> (w429:string[])
                      n222 = node-c288(i64 2000 ("Start")) -> ()  [unwired: 1 out]
                      n223 = call-poly <vilib>:"Write Delimited Spreadsheet.vi"("file path (dialog if empty)"=w417, "format (%s)"="%.6f" ("format (%.3f)"), "1D data"=w429, "append to file? (new file:F)"=TRUE, "delimiter (\\t)"="," ("delimiter (\\t)")) -> ()  [unwired: 9 in, 2 out]
                    }
                    frame #5 {
                      w454 = u16 4 items=["A", "B", "C", "D", "E", "F"]
                      w462 = u16 5 items=["A", "B", "C", "D", "E", "F"]
                      w463 = i16 7 ("precision (6)")
                      n224 = node-c288() -> ()  [unwired: 1 in, 1 out]
                      n225 = local read "Meas. Data (for active device)"() -> (w460:T3)
                      n226 = Unbundle(w460) -> ("Absolute Pressure"=w480:dbl, "Temperature"=w476:dbl, "Volumetric Flow"=w467:dbl, "Mass Flow"=w477:dbl, "Setpoint"=w478:dbl)  [unwired: 10 out]
                      n227 = local read "FSP"() -> (w455:dbl)
                      n228 = Number To Fractional String(number=w480, precision (6)=w463) -> (F-format string=w475:string)  [unwired: 2 in]
                      n229 = Number To Fractional String(number=w476, precision (6)=w463) -> (F-format string=w474:string)  [unwired: 2 in]
                      n230 = Number To Fractional String(number=w467, precision (6)=w463) -> (F-format string=w473:string)  [unwired: 2 in]
                      n231 = Number To Fractional String(number=w477, precision (6)=w463) -> (F-format string=w472:string)  [unwired: 2 in]
                      n232 = Number To Fractional String(number=w478, precision (6)=w463) -> (F-format string=w471:string)  [unwired: 2 in]
                      n233 = local read "Z"() -> (w459:dbl[])
                      n234 = local read "T_SCh"() -> (w453:string[])
                      n235 = local read "Iter_#"() -> (w451:string)
                      n236 = local read "V_D"() -> (w450:string)
                      n237 = local read "V_H"() -> (w449:string)
                      n238 = local read "Iter_Duration"() -> (w448:string)
                      n239 = Replace Array Subset(array=w459, new element #1=w462, index #1=1 ("index"), new element #2=w455, index #2=0 ("index")) -> (w458:dbl[])
                      n240 = Number To Fractional String(number=w454, precision (6)=w463) -> (F-format string=w479:string)  [unwired: 2 in]
                      n241 = Get Date/Time In Seconds() -> (seconds since 1Jan1904=w466:timestamp)
                      n242 = Get Date/Time String(seconds (now)=w466, want seconds? (F)=TRUE) -> (date string=w465:string, time string=w481:string)  [unwired: 1 in]
                      n243 = local write "Z"(w458) -> ()
                      n244 = Build Array (concatenate)(w465, w481, w479, w475, w474, w473, w472, w471, w453, w451, w450, w449, w448) -> (w468:string[])
                      n245 = call-poly <vilib>:"Write Delimited Spreadsheet.vi"("file path (dialog if empty)"=w457, "format (%s)"="%.6f" ("format (%.3f)"), "1D data"=w468, "append to file? (new file:F)"=TRUE, "delimiter (\\t)"="," ("delimiter (\\t)")) -> ()  [unwired: 9 in, 2 out]
                      n246 = node-c288(i64 2000 ("Start")) -> ()  [unwired: 1 out]
                    }
                    frame #6 {
                      n247 = node-c288() -> ()  [unwired: 1 in, 1 out]
                      n248 = local read "read count"() -> (w493:dbl)
                      n249 = local read "N_read"() -> (w491:i32)
                      n250 = call <extravilib>:"Read.vi"("channel"=w489) -> ("element"=w488:bool)  [unwired: 1 in, 1 out]
                      n251 = Subtract(x=w493, y=2.0) -> (x-y=w492:dbl)
                      n252 = node-c288() -> ()  [unwired: 1 in, 1 out]
                      n253 = Equal?(x=w491, y=w492) -> (x = y?=w490:bool)
                      n254 = Or(x=w490, y=w488) -> (x .or. y?=w487:bool)
                    }
                  }
                }
                n255 = node-c288() -> ()  [unwired: 1 in, 1 out]
                n256 = node-c288() -> ()  [unwired: 1 in, 1 out]
              }
              n257 = local read "Hold Time [min]"() -> (w220:dbl)
              n258 = Multiply(x=w220, y=60000.0) -> (x*y=w219:dbl)
              n259 = Subtract(x=w219, y=12000.0) -> (x-y=w216:dbl)
              n260 = Divide(x=w216, y=w217) -> (x/y=→"N_i_read":dbl)
              n261 = Equal?(x=w224, y=0.0) -> (x = y?=w226:bool)
              n262 = call <extravilib>:"Read.vi"("channel"=w214) -> ("element"=w225:bool)  [unwired: 1 in, 1 out]
              n263 = Or(x=w226, y=w225) -> (x .or. y?=w223:bool)
              n264 = node-c288(w229) -> ()  [unwired: 1 out]
              "read count" <- w217
            }
            n265 = node-c288() -> ()  [unwired: 1 in, 1 out]
          }
        }
      }
      n266 = node-c288() -> ()  [unwired: 1 in, 1 out]
      n267 = node-c288() -> ()  [unwired: 1 in, 1 out]
    }
    n268 = Unbundle("COM Port Settings") -> ("Baud Rate"=w34:T9, "VISA Sesssion In"=w33:refnum<visa-resource-name>)
    n269 = Bundle(cluster=T4 {"Unit ID"="A", "Baud Rate"=enum."19200", "VISA Sesssion In"="COM1"} ("Communication Settings"), "Baud Rate"=w34, "VISA Sesssion In"=w33) -> (w32:T4)  [unwired: 1 in]
    n270 = Cluster To Array(cluster="Device ID's \nto Include:") -> (array=w28:bool[])
    n271 = call "COM Port Initialization.vi"("error in (no error)"=errorcluster {"status"=FALSE, "code"=0, "source"=""}, "Communication Settings"=w32) -> ("error out"=w25:errorcluster, "VISA Session Out"=w24:refnum<visa-resource-name>)  [unwired: 8 in]
    n272 = for {
      N: 6 -> [_]
      tunnel: "ABCDEF" -> [w534]
      tunnel: w28 -> [w527] mode=indexing
      shift-right: [w526] -> _
      shift-left: u16 0 ("length (rest)") -> [w532]
      shift-right: [w531] -> w22
      shift-left: cluster{string, u16}[] [] -> [w530]
      tunnel: w25 -> [w525]
      tunnel: w24 -> [w524]
      tunnel: [w525] -> w15
      tunnel: [w524] -> w23
      i -> [w533]
      # "Generate array of Device ID's, with sequential ID's"
      n273 = Equal?(x=w527, y=TRUE) -> (x = y?=w529:bool)
      n274 = case shown="True" w529 {
        tunnel: w534 -> [_ w545]
        tunnel: w533 -> [_ w544]
        tunnel: w532 -> [w535 w537]
        tunnel: [w536 w540] -> w531
        tunnel: w530 -> [w536 w538]
        tunnel: [w535 w541] -> w526
        frame False {
          # "ID was not included"
        }
        frame True {
          # "ID was included"
          n275 = String Subset(string=w545, offset (0)=w544, length (rest)=1 ("length (rest)")) -> (substring=w542:string)
          n276 = Bundle(w542, "length (rest)"=w537) -> (w539:cluster{string, "length (rest)":u16})  [unwired: 1 in]
          n277 = Increment(x=w537) -> (x+1=w541:u16)
          n278 = Build Array (concatenate)(w538, w539) -> (w540:cluster{string, "length (rest)":u16}[])
        }
      }
    }
    n279 = property on="Active Device" class="Ring (strict)"(error in=w15, "StringsAndValues[]"=w22) -> (error out=w14:errorcluster)  [unwired: 1 in, 1 out]
    n280 = for {
      tunnel: w23 -> [w522]
      tunnel: [w519] -> w19
      tunnel: w14 -> [w523]
      tunnel: [w518] -> w18
      tunnel: w22 -> [w520] mode=indexing
      tunnel: [w521] -> w21 mode=indexing
      tunnel: [w511] -> w20 mode=indexing
      tunnel: [w517] -> w17 mode=indexing
      tunnel: [nan ("Setpoint")] -> w16 mode=indexing
      tunnel: [w510] -> w13 mode=indexing
      # "Get measurement formats, unit ID's and the controller info"
      n281 = Unbundle(w520) -> (w511:string)  [unwired: 1 out]
      n282 = call "Read Measurement Format.vi"("Unit ID (A)"=w511, "error in"=w523, "VISA Session In"=w522) -> ("error out"=w514:errorcluster, "Data Frame Format"=w521:T10, "VISA Session Out"=w515:refnum<visa-resource-name>)  [unwired: 6 in]
      n283 = property on="Active Device" class="Ring (strict)" props=["Value"]() -> ()  [unwired: 2 in, 3 out]
      n284 = call "Read Software Version.vi"("Unit ID (A)"=w511, "error in"=w514, "VISA Session In"=w515) -> ("error out"=w513:errorcluster, "Software Version"=w510:u8, "VISA Session Out"=w512:refnum<visa-resource-name>)  [unwired: 6 in]
      n285 = call "Read Controller Info.vi"("Unit ID (A)"=w511, "error in"=w513, "Software Version"=w510, "VISA Session In"=w512) -> ("error out"=w518:errorcluster, "Controller Info out"=w517:T11, "VISA Session Out"=w519:refnum<visa-resource-name>)  [unwired: 4 in, 1 out]
    }
    n286 = while {
      shift-right: [w582] -> _
      shift-left: 0.0 ("Set Start Time (s)") -> [w585]
      shift-right: [w566] -> w37
      shift-left: w18 -> [w584]
      shift-right: [w567] -> w38
      shift-left: w19 -> [w583]
      tunnel: w20 -> [w559]
      shift-right: [w570] -> _
      shift-left: w21 -> [w577]
      shift-right: [w565] -> _
      shift-left: w17 -> [w563]
      shift-right: [w561] -> _
      shift-left: w16 -> [w560]
      shift-right: [w555] -> _
      shift-left: w13 -> [w555]
      tunnel: w9 -> [w553]
      stop <- w554 stop-if-true
      # "Set minimum time\nbetween loops"
      # "Acquire data for every device ID included at the requested data rate, then display only the selected device's data"
      n287 = call "Elapsed Time"("Set Start Time (s)"=w585) -> ("Get Start Time (s)"=w582:dbl, "Elapsed Time (s)"=w579:dbl)  [unwired: 11 in, 6 out]
      n288 = Wait (ms)(milliseconds to wait="Minimum time between \nreadings [ms] (all units)") -> ()  [unwired: 1 out]
      n289 = for {
        shift-right: [w614] -> w576
        shift-left: w584 -> [w617]
        shift-right: [w615] -> w575
        shift-left: w583 -> [w616]
        tunnel: w577 -> [w611] mode=indexing
        tunnel: w559 -> [w610] mode=indexing
        tunnel: [w609] -> w574 mode=indexing
        tunnel: [w608] -> w573 mode=indexing
        tunnel: [w607] -> w572 mode=indexing
        tunnel: [w606] -> w571 mode=indexing
        tunnel: [w605] -> w570 mode=indexing
        # "Acquire data for each device"
        n290 = call "Read Measurements.vi"("error in"=w617, "Data Frame Format In"=w611, "Unit ID (A)"=w610, "VISA Session In"=w616) -> ("error out"=w614:errorcluster, "Data Frame Format Out"=w605:T10, "Data Cluster"=w608:T3, "VISA Session Out"=w615:refnum<visa-resource-name>, "Unknown Dataframe Info"=w613:bool, "Error/Overrange/Unknown String"=w607:string, "Error Present"=w612:bool, "Range Exceeded"=w606:bool)
        n291 = Or(x=w613, y=w612) -> (x .or. y?=w609:bool)
      }
      n292 = Multiply(x=1000.0 ("y"), y=w579) -> (x*y=→"Elapsed Time [ms]\n(all units)":dbl)
      n293 = Reciprocal(x=w579) -> ()  [unwired: 1 out]
      n294 = local read "Z"() -> (w549:dbl[])
      n295 = Index Array(array=w549, index=1 ("index (row)")) -> (element=w547:dbl)
      "Active Device" <- w547
      n296 = To Long Integer(number=w547) -> (32bit integer=w557:i32)
      n297 = for {
        tunnel: w576 -> [w588]
        tunnel: [w587] -> w568
        tunnel: w575 -> [w589]
        tunnel: [w586] -> w569
        tunnel: w574 -> [w594] mode=indexing
        tunnel: w557 -> [w596]
        tunnel: w573 -> [w593] mode=indexing
        tunnel: w572 -> [w592] mode=indexing
        tunnel: w571 -> [w591] mode=indexing
        i -> [w595]
        # "Iterate over all sets of data, only display the one selected"
        n298 = Equal?(x=w596, y=w595) -> (x = y?=w590:bool)
        n299 = case shown="True" w590 {
          tunnel: w594 -> [_ w604]
          tunnel: w593 -> [_ w599]
          tunnel: w592 -> [_ w603]
          tunnel: w591 -> [_ w602]
          tunnel: w589 -> [w598 w600]
          tunnel: w588 -> [w597 w601]
          tunnel: [w597 w601] -> w587
          tunnel: [w598 w600] -> w586
          frame False {
            # "Do nothing"
          }
          frame True {
            # "Display data"
            "Range Exceeded" <- w602
            "Error Present" <- w604
            "Error Text" <- w603
            "Meas. Data (for active device)" <- w599
          }
        }
      }
      n300 = Index Array(array=w555, index=w557) -> (element=w556:u8)
      n301 = local read "Z"() -> (w552:dbl[])
      n302 = Index Array(array=w559, index=w557) -> (element=w558:string)
      n303 = Index Array(array=w563, index=w557) -> (element=w562:T11)
      n304 = Index Array(array=w560, index=w557) -> (element=w546:dbl)
      n305 = Index Array(array=w552, index=0) -> (element=w550:dbl)
      n306 = call "Write SetPoint_no prev.vi"("Setpoint"=w550, "Previous Setpoint"=w546, "Unit ID (A)"=w558, "error in"=w568, "Software Version"=w556, "Controller Info out"=w562, "VISA Session In"=w569) -> ("error out"=w566:errorcluster, "Controller Info out"=w564:T11, "VISA Session Out"=w567:refnum<visa-resource-name>)  [unwired: 1 in, 1 out]
      n307 = Replace Array Subset(array=w560, new element=w550, index=w557) -> (w561:dbl[])
      n308 = Replace Array Subset(array=w563, new element=w564, index=w557) -> (w565:T12)
      n309 = call <extravilib>:"Read.vi"("channel"=w553) -> ("element"=w554:bool)  [unwired: 1 in, 1 out]
    }
    n310 = call-poly <vilib>:"Write Delimited Spreadsheet.vi"("file path (dialog if empty)"="Write File", "1D data"=string[] ["Date", "Time [hh:mm:ss]", "Device ID", "Abs_P_MFC [psi]", "T_MFC [C]", "Volume Flow [LPM]", "Mass Flow [SLPM]", "SP_MFC [LPM]", "T_SCh", "Iter_#", "V_D", "V_H", "Iter_Duration", ""], "append to file? (new file:F)"=TRUE, "delimiter (\\t)"="," ("delimiter (\\t)")) -> ()  [unwired: 10 in, 2 out]
    n311 = VISA Close(VISA resource name=w38, error in (no error)=w37) -> (error out=w39:errorcluster)
    n312 = call <vilib>:"Simple Error Handler.vi"("error in (no error)"=w39) -> ()  [unwired: 4 in, 5 out]
    n313 = Initialize Array(0.0 ("element"), 2 ("dimension size")) -> (→"Z":dbl[])
    n314 = while "Hold Setpoints" {
      tunnel: w9 -> [w50]
      stop <- w51 stop-if-true
      n315 = call-poly <vilib>:"Read Delimited Spreadsheet.vi"("file path (dialog if empty)"="Read File", "start of read offset (chars.:0)"=0, "delimiter (\\t)"="," ("delimiter (\\t)")) -> ("all rows"=w46:dbl[][])  [unwired: 7 in, 5 out]
      "all rows" <- w46
      n316 = Array Subset(array=w46, index (row)="Start From:") -> (w44:dbl[][])  [unwired: 3 in]
      "Setpoints" <- w44
      n317 = call <extravilib>:"Read.vi"("channel"=w50) -> ("element"=w51:bool)  [unwired: 1 in, 1 out]
      n318 = Array Size(array=w44) -> (size(s)=w53:i32[])
      n319 = Index Array(array=w53, index=0) -> (element=→"len_SP":i32)
    }
    n320 = node-c288(w42) -> ()  [unwired: 1 out]
  }
